vi "GUI_TEST.vi"() -> ()   [LabVIEW 2024]
uses:
  <vilib>/Utility/config.llb/Read Key (String).vi
  Variables/Download Confrigurations.vi
  <vilib>/Utility/config.llb/NI_LVConfig.lvlib
panel:
  out "error out":errorcluster
  in  "error in":errorcluster
  in  "Main Tab":enum32{"MAIN"}(tab)
  out "INSTR":bool
  in  "Operation Tab":enum32{"LOGIN"}(tab)
  in  "CHANGE PASSWORD":bool
  in  "FORGET PASSWORD":bool
  in  "RESET PASSWORD":bool
  in  "LOGIN-START":bool
  in  "PASSWORD":string
  in  "USER ID":string
  out "DB":bool
  in  "EXIT":bool
  in  "LOG-OUT":bool
  in  "Settings Button":bool
  in  "ABORT TEST":bool
  in  "START TEST":bool
  in  "LOGIN BUTTON":bool
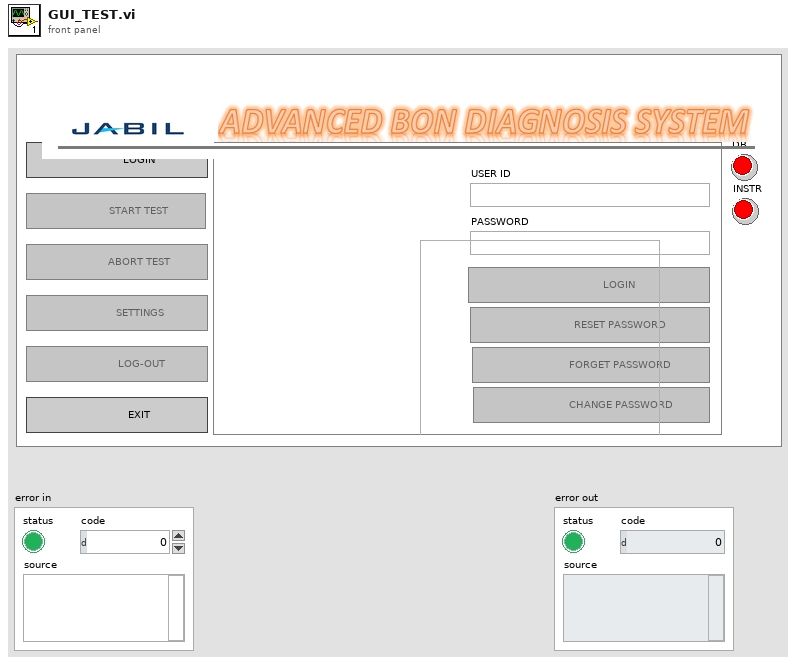
[diagram p1: front panel]
types:
  T1 = enum8{"Enabled", "Disabled", "Disabled and Grayed Out"}
  T2 = typedef "NI_LVConfig.lvlib/Config Data RefNum.ctl" = refnum<k1>
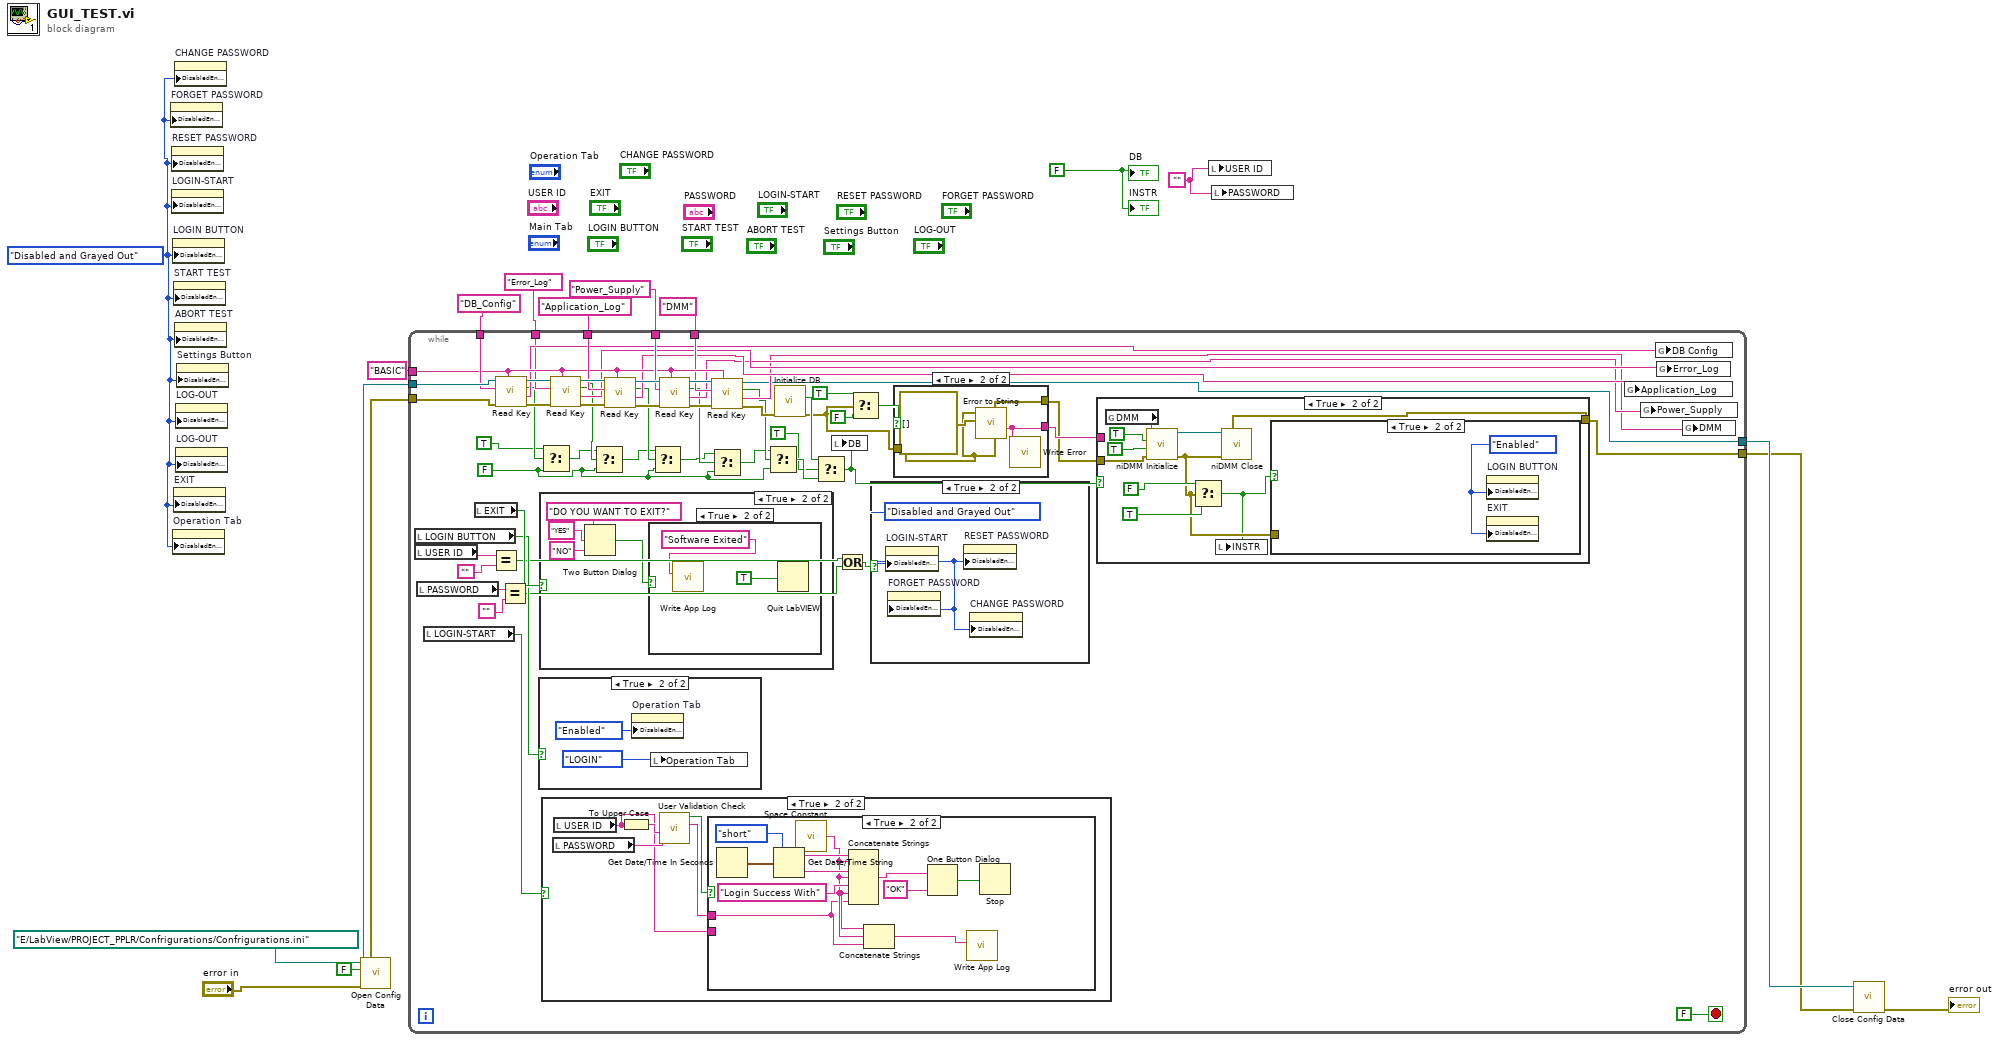
[diagram p0: block diagram]
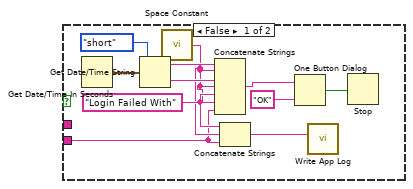
[diagram p3: hidden frame]
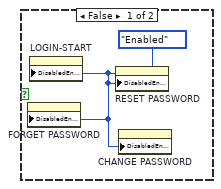
[diagram p4: hidden frame]
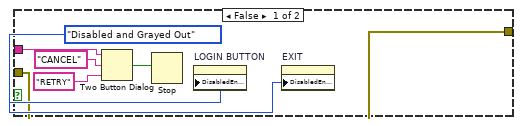
[diagram p8: hidden frame]
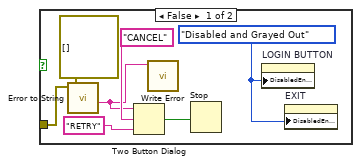
[diagram p9: hidden frame]
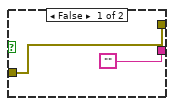
[diagram p10: hidden frame]
diagram:
  w1 = ""
  w2 = FALSE
  w4 = T1."Disabled and Grayed Out" ("Disabled")
  n1 = property on="FORGET PASSWORD" class="Bool (strict)"("DisabledEnum"=w4) -> ()  [unwired: 2 in, 2 out]
  n2 = property on="RESET PASSWORD" class="Bool (strict)"("DisabledEnum"=w4) -> ()  [unwired: 2 in, 2 out]
  n3 = property on="LOGIN-START" class="Bool (strict)"("DisabledEnum"=w4) -> ()  [unwired: 2 in, 2 out]
  n4 = property on="LOGIN BUTTON" class="Bool (strict)"("DisabledEnum"=w4) -> ()  [unwired: 2 in, 2 out]
  n5 = property on="Operation Tab" class="TabCtl (strict)"("DisabledEnum"=w4) -> ()  [unwired: 2 in, 2 out]
  n6 = property on="START TEST" class="Bool (strict)"("DisabledEnum"=w4) -> ()  [unwired: 2 in, 2 out]
  n7 = property on="EXIT" class="Bool (strict)"("DisabledEnum"=w4) -> ()  [unwired: 2 in, 2 out]
  n8 = property on="CHANGE PASSWORD" class="Bool (strict)"("DisabledEnum"=w4) -> ()  [unwired: 2 in, 2 out]
  n9 = property on="ABORT TEST" class="Bool (strict)"("DisabledEnum"=w4) -> ()  [unwired: 2 in, 2 out]
  n10 = property on="LOG-OUT" class="Bool (strict)"("DisabledEnum"=w4) -> ()  [unwired: 2 in, 2 out]
  n11 = property on="LOG-OUT" class="Bool (strict)"("DisabledEnum"=w4) -> ()  [unwired: 2 in, 2 out]
  n12 = property on="Settings Button" class="Bool (strict)"("DisabledEnum"=w4) -> ()  [unwired: 2 in, 2 out]
  n13 = call <vilib>:"Open Config Data.vi"("error in (no error)"="error in", "create file if necessary (T)"=FALSE, "configuration file path"=path "E:/LabView/PROJECT_PPLR/Confrigurations/Confrigurations.ini") -> ("error out"=w13:errorcluster, "refnum"=w14:T2)  [unwired: 6 in, 1 out]
  n14 = while {
    tunnel: w14 -> [w72]
    tunnel: w13 -> [w71]
    tunnel: "BASIC" ("section") -> [w59]
    tunnel: "DB_Config" ("key") -> [w70]
    tunnel: "Error_Log" ("default value") -> [w52]
    tunnel: "Application_Log" ("key") -> [w65]
    tunnel: "Power_Supply" ("key") -> [w62]
    tunnel: "DMM" ("key") -> [w58]
    tunnel: [w51] -> w5
    tunnel: [w28] -> w3
    stop <- FALSE stop-if-true
    w39 = FALSE
    n15 = local read "LOGIN BUTTON"() -> (w26:bool)
    n16 = local read "USER ID"() -> (w23:string)
    n17 = local read "PASSWORD"() -> (w20:string)
    n18 = local read "LOGIN-START"() -> (w18:bool)
    n19 = local read "EXIT"() -> (w27:bool)
    n20 = Equal?(x=w23, y="") -> (x = y?=w22:bool)
    n21 = call-poly <vilib>:"Read Key.vi"("section"=w59, "error in (no error)"=w71, "key"=w70, "refnum"=w72) -> ("error out"=w68:errorcluster, "value"=w57:string, "found?"=w49:bool, "refnum out"=w69:T2)  [unwired: 4 in]
    n22 = Equal?(x=w20, y="") -> (x = y?=w19:bool)
    n23 = case shown="True" w26 {
      frame False {
      }
      frame True {
        n24 = property on="Operation Tab" class="TabCtl (strict)"("DisabledEnum"=T1."Enabled" ("Disabled")) -> ()  [unwired: 2 in, 2 out]
        n25 = local write "Operation Tab"(enum32{"LOGIN", "Page 2"}."LOGIN" ("Operation Tab")) -> ()
      }
    }
    n26 = case shown="True" w27 {
      frame False {
      }
      frame True {
        n27 = Two Button Dialog(message="DO YOU WANT TO EXIT?", 1:"NO" ("F button name (\"Cancel\")"), 2:"YES" ("T button name (\"OK\")")) -> (T button?=w105:bool)
        n28 = case shown="True" w105 {
          frame False {
          }
          frame True {
            n29 = call "Write App Log.vi"("String To Write"="Software Exited") -> ()  [unwired: 9 in, 2 out]
            n30 = Quit LabVIEW(quit? (T)=TRUE) -> ()
          }
        }
      }
    }
    n31 = Select(t=TRUE, s=w49, f=w39) -> (s? t:f=w46:bool)
    n32 = case shown="True" w18 {
      frame False {
      }
      frame True {
        n33 = local read "PASSWORD"() -> (w77:string)
        n34 = local read "USER ID"() -> (w74:string)
        n35 = To Upper Case(1:w74) -> (0:w78:string)
        n36 = call "User Validation Check.vi"("Password"=w77, "UserName"=w78) -> ("FoundUserName"=w75:string, "MatchFound?"=w76:bool)  [unwired: 7 in, 1 out]
        n37 = case shown="True" w76 {
          tunnel: w75 -> [_ w91]
          tunnel: w74 -> [w80 _]
          frame False {
            w82 = "Login Failed With"
            n38 = Get Date/Time In Seconds() -> (seconds since 1Jan1904=w89:timestamp)
            n39 = Get Date/Time String(date format (0)=enum16{"short", "long", "abbreviated"}."short", seconds (now)=w89) -> (date string=w87:string, time string=w86:string)  [unwired: 1 in]
            n40 = call <vilib>:"Space Constant.vi"() -> ("String"=w81:string)
            n41 = Concatenate Strings(w87, w81, w86, w81, w82, w81, w80) -> (w83:string)
            n42 = Concatenate Strings(w82, w81, w80) -> (w79:string)
            n43 = One Button Dialog(message=w83, button name ("OK")="OK") -> (true=w84:bool)
            n44 = call "Write App Log.vi"("String To Write"=w79) -> ()  [unwired: 9 in, 2 out]
            n45 = Stop(stop? (T)=w84) -> ()
          }
          frame True {
            n46 = Get Date/Time In Seconds() -> (seconds since 1Jan1904=w100:timestamp)
            n47 = Get Date/Time String(date format (0)=enum16{"short", "long", "abbreviated"}."short", seconds (now)=w100) -> (date string=w98:string, time string=w97:string)  [unwired: 1 in]
            n48 = call <vilib>:"Space Constant.vi"() -> ("String"=w92:string)
            n49 = Concatenate Strings(w98, w92, w97, w92, "Login Success With", w92, w91) -> (w93:string)
            n50 = Concatenate Strings(w92, w92, w91) -> (w90:string)
            n51 = One Button Dialog(message=w93, button name ("OK")="OK") -> (true=w94:bool)
            n52 = call "Write App Log.vi"("String To Write"=w90) -> ()  [unwired: 9 in, 2 out]
            n53 = Stop(stop? (T)=w94) -> ()
          }
        }
      }
    }
    n54 = call-poly <vilib>:"Read Key.vi"("section"=w59, "error in (no error)"=w68, "key"=w52, "refnum"=w69) -> ("error out"=w66:errorcluster, "value"=w56:string, "found?"=w47:bool, "refnum out"=w67:T2)  [unwired: 4 in]
    n55 = Select(t=w46, s=w47, f=w39) -> (s? t:f=w44:bool)
    n56 = call-poly <vilib>:"Read Key.vi"("section"=w59, "error in (no error)"=w66, "key"=w65, "refnum"=w67) -> ("error out"=w63:errorcluster, "value"=w55:string, "found?"=w45:bool, "refnum out"=w64:T2)  [unwired: 4 in]
    n57 = Select(t=w44, s=w45, f=w39) -> (s? t:f=w42:bool)
    n58 = call-poly <vilib>:"Read Key.vi"("section"=w59, "error in (no error)"=w63, "key"=w62, "refnum"=w64) -> ("error out"=w60:errorcluster, "value"=w54:string, "found?"=w43:bool, "refnum out"=w61:T2)  [unwired: 4 in]
    n59 = call-poly <vilib>:"Read Key.vi"("section"=w59, "error in (no error)"=w60, "key"=w58, "refnum"=w61) -> ("error out"=w50:errorcluster, "value"=w53:string, "found?"=w41:bool, "refnum out"=w51:T2)  [unwired: 4 in]
    n60 = Select(t=w42, s=w43, f=w39) -> (s? t:f=w40:bool)
    n61 = Select(t=w40, s=w41, f=w39) -> (s? t:f=w37:bool)
    n62 = call "Initialize DB.vi"("error in (no error)"=w50) -> ("error out"=w32:errorcluster, "DB Connected?"=w38:bool)  [unwired: 8 in, 1 out]
    n63 = Select(t=w38, s=TRUE, f=w37) -> (s? t:f=w31:bool)
    n64 = local write "DB"(w31) -> ()
    n65 = Or(x=w22, y=w19) -> (x .or. y?=w25:bool)
    n66 = Select(t=TRUE, s=w32, f=FALSE) -> (s? t:f=w33:bool)
    n67 = case shown="True" w25 {
      frame False {
        w101 = T1."Enabled" ("Disabled")
        n68 = property on="FORGET PASSWORD" class="Bool (strict)"("DisabledEnum"=w101) -> ()  [unwired: 2 in, 2 out]
        n69 = property on="LOGIN-START" class="Bool (strict)"("DisabledEnum"=w101) -> ()  [unwired: 2 in, 2 out]
        n70 = property on="RESET PASSWORD" class="Bool (strict)"("DisabledEnum"=w101) -> ()  [unwired: 2 in, 2 out]
        n71 = property on="CHANGE PASSWORD" class="Bool (strict)"("DisabledEnum"=w101) -> ()  [unwired: 2 in, 2 out]
      }
      frame True {
        w102 = T1."Disabled and Grayed Out" ("Disabled")
        n72 = property on="LOGIN-START" class="Bool (strict)"("DisabledEnum"=w102) -> ()  [unwired: 2 in, 2 out]
        n73 = property on="FORGET PASSWORD" class="Bool (strict)"("DisabledEnum"=w102) -> ()  [unwired: 2 in, 2 out]
        n74 = property on="RESET PASSWORD" class="Bool (strict)"("DisabledEnum"=w102) -> ()  [unwired: 2 in, 2 out]
        n75 = property on="CHANGE PASSWORD" class="Bool (strict)"("DisabledEnum"=w102) -> ()  [unwired: 2 in, 2 out]
      }
    }
    n76 = case shown="True" w33 {
      tunnel: w32 -> [w136 w138]
      tunnel: [w136 w138] -> w29
      tunnel: ["" w137] -> w30
      frame False {
      }
      frame True {
        n77 = call "Error to String.vi"("Error Array"=errorcluster[] [], "Error In"=w138) -> ("Error String"=w137:string)  [unwired: 4 in, 1 out]
        n78 = call "Write Error.vi"("Error String"=w137) -> ()  [unwired: 8 in, 3 out]
      }
    }
    n79 = case shown="True" w31 {
      tunnel: w30 -> [w116 _]
      tunnel: w29 -> [w111 w123]
      tunnel: [w111 w119] -> w28
      frame False {
        w114 = T1."Disabled and Grayed Out" ("Disabled")
        n80 = Two Button Dialog(message=w116, 1:"RETRY" ("F button name (\"Cancel\")"), 2:"CANCEL" ("T button name (\"OK\")")) -> (T button?=w112:bool)
        n81 = Stop(stop? (T)=w112) -> ()
        n82 = property on="LOGIN BUTTON" class="Bool (strict)"("DisabledEnum"=w114) -> ()  [unwired: 2 in, 2 out]
        n83 = property on="EXIT" class="Bool (strict)"("DisabledEnum"=w114) -> ()  [unwired: 2 in, 2 out]
      }
      frame True {
        n84 = global read "Download Confrigurations.vi" "DMM"() -> (w126:string)
        n85 = call <instrlib>:"niDMM Initialize.vi"("error in (no error)"=w123, "Reset"=TRUE, "ID Query"=TRUE, "Instrument Descriptor"=w126) -> ("error out"=w118:errorcluster, "instrument handle out"=w122:refnum<k15>)  [unwired: 6 in]
        n86 = Select(t=FALSE, s=w118, f=TRUE) -> (s? t:f=w117:bool)
        n87 = local write "INSTR"(w117) -> ()
        n88 = call <instrlib>:"niDMM Close.vi"("error in (no error)"=w118, "instrument handle"=w122) -> ("error out"=w119:errorcluster)  [unwired: 9 in]
        n89 = case shown="True" w117 {
          tunnel: w118 -> [w131 _]
          frame False {
            w133 = T1."Disabled and Grayed Out" ("Disabled")
            n90 = call "Error to String.vi"("Error Array"=errorcluster[] [], "Error In"=w131) -> ("Error String"=w127:string)  [unwired: 4 in, 1 out]
            n91 = Two Button Dialog(message=w127, 1:"RETRY" ("F button name (\"Cancel\")"), 2:"CANCEL" ("T button name (\"OK\")")) -> (T button?=w128:bool)
            n92 = call "Write Error.vi"("Error String"=w127) -> ()  [unwired: 8 in, 3 out]
            n93 = Stop(stop? (T)=w128) -> ()
            n94 = property on="LOGIN BUTTON" class="Bool (strict)"("DisabledEnum"=w133) -> ()  [unwired: 2 in, 2 out]
            n95 = property on="EXIT" class="Bool (strict)"("DisabledEnum"=w133) -> ()  [unwired: 2 in, 2 out]
          }
          frame True {
            w134 = T1."Enabled" ("Disabled")
            n96 = property on="LOGIN BUTTON" class="Bool (strict)"("DisabledEnum"=w134) -> ()  [unwired: 2 in, 2 out]
            n97 = property on="EXIT" class="Bool (strict)"("DisabledEnum"=w134) -> ()  [unwired: 2 in, 2 out]
          }
        }
      }
    }
    n98 = global write "Download Confrigurations.vi" "Application_Log"(w55) -> ()
    n99 = global write "Download Confrigurations.vi" "Power_Supply"(w54) -> ()
    n100 = global write "Download Confrigurations.vi" "DB Config"(w57) -> ()
    n101 = global write "Download Confrigurations.vi" "Error_Log"(w56) -> ()
    n102 = global write "Download Confrigurations.vi" "DMM"(w53) -> ()
  }
  n103 = local write "USER ID"(w1) -> ()
  n104 = local write "PASSWORD"(w1) -> ()
  n105 = call <vilib>:"Close Config Data.vi"("error in (no error)"=w3, "refnum"=w5) -> ("error out"=→"error out":errorcluster)  [unwired: 8 in, 1 out]
  "DB" <- w2
  "INSTR" <- w2
